vi "Demo - GNU Octave Terminal.vi"() -> ()   [LabVIEW 2013, in "GOLPI library.lvlib"]
uses:
  GOLPI library.lvlib
  LV Process.lvlibp/Pipe Handle.ctl
  LV Process.lvlibp
panel:
  out "bytes remaining":i32
  in  "quit":bool
  out "GNU Octave running":bool
  out "read buffer":string
  in  "command buffer":string
  in  "command":bool
  out "objects after start":refnum<vi>[](array[refnum])
  out "objects before start":refnum<vi>[](array[refnum])
  in  "stop":bool
  out "error":errorcluster
  out "octave pipe":T1
  in  "start":bool
  in  "Octave binary directory":path=path "C:/Program Files/Octave-3.6.2/bin"
  in  "Working directory":path=path "C:/"
  out "exit code":i32
  out "GNU Octave version":string
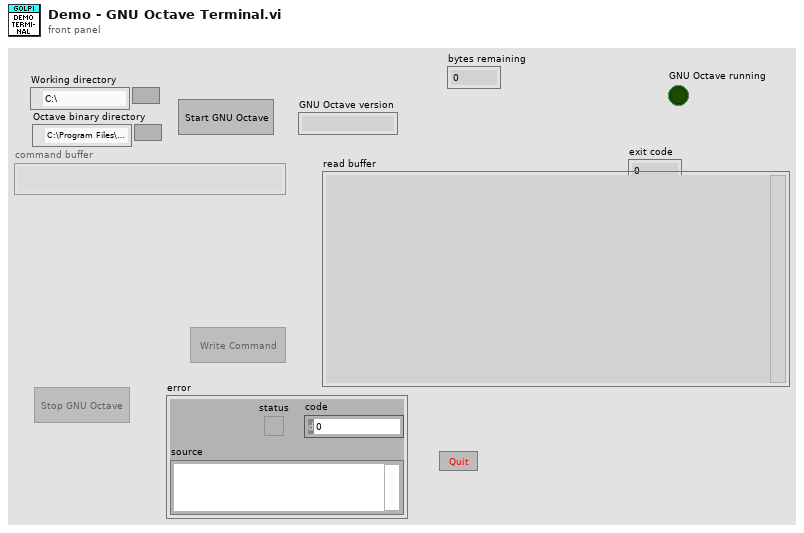
[diagram p1: front panel]
types:
  T1 = typedef "LV Process.lvlibp/Pipe Handle.ctl" = cluster{"lv_proc.dll file path":path, "process instance handle":u32[]}
  T2 = enum8{"Enabled", "Disabled", "Disabled and Grayed Out"}
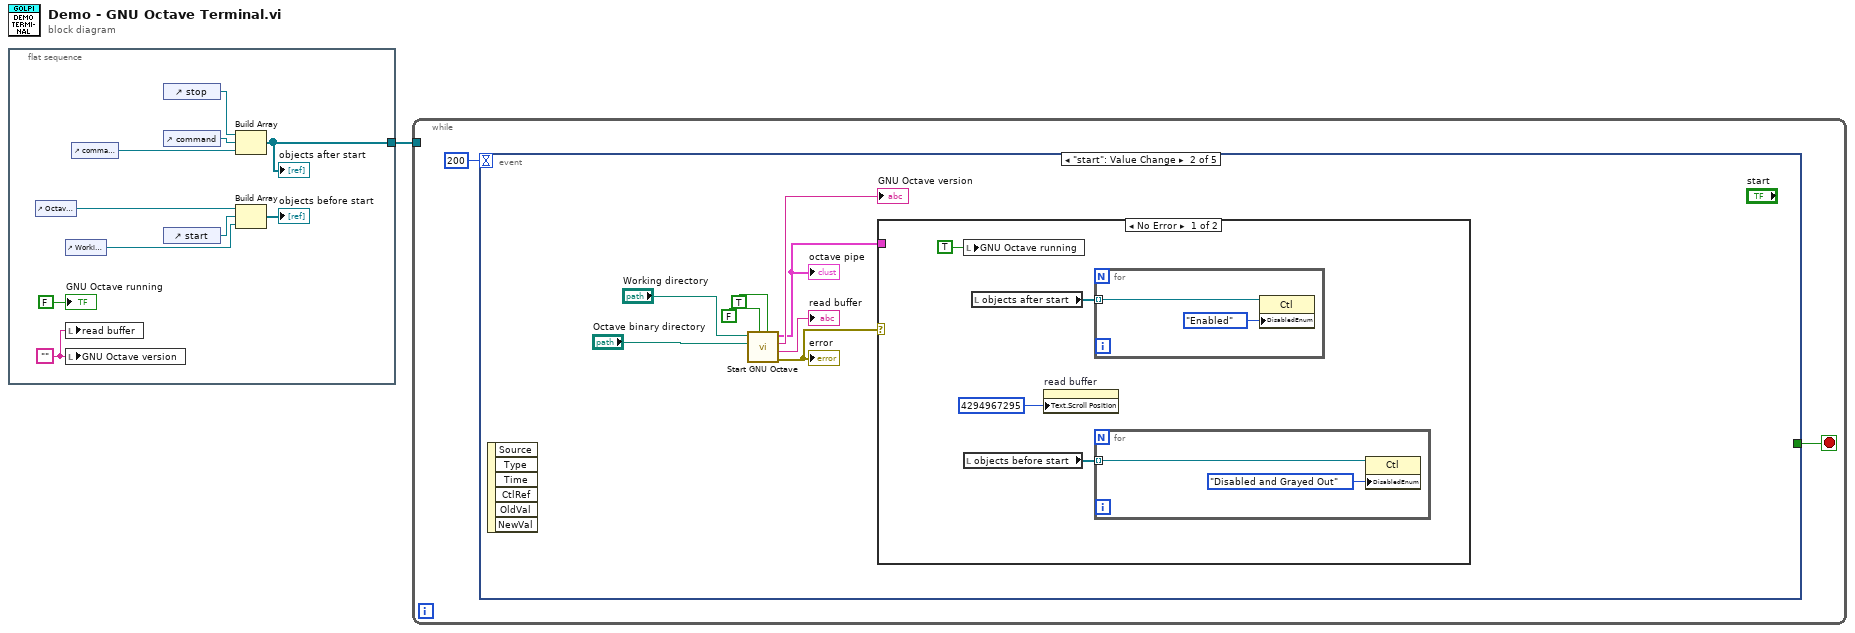
[diagram p0: block diagram]
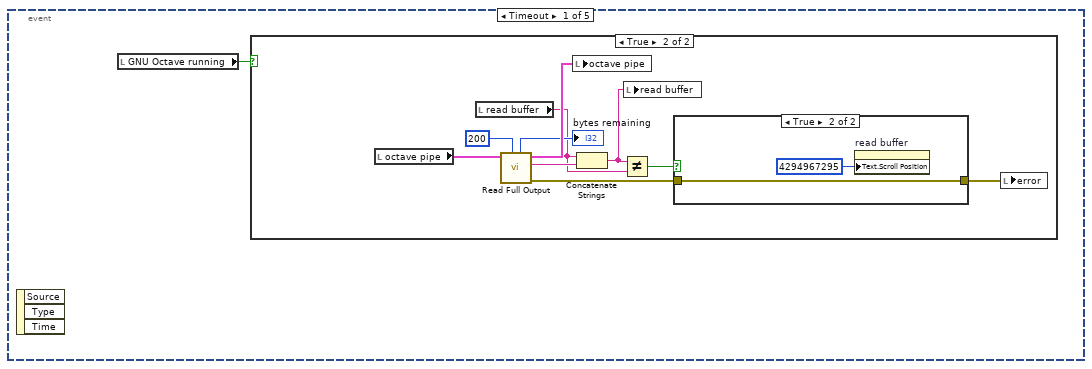
[diagram p2: hidden frame]
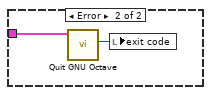
[diagram p5: hidden frame]
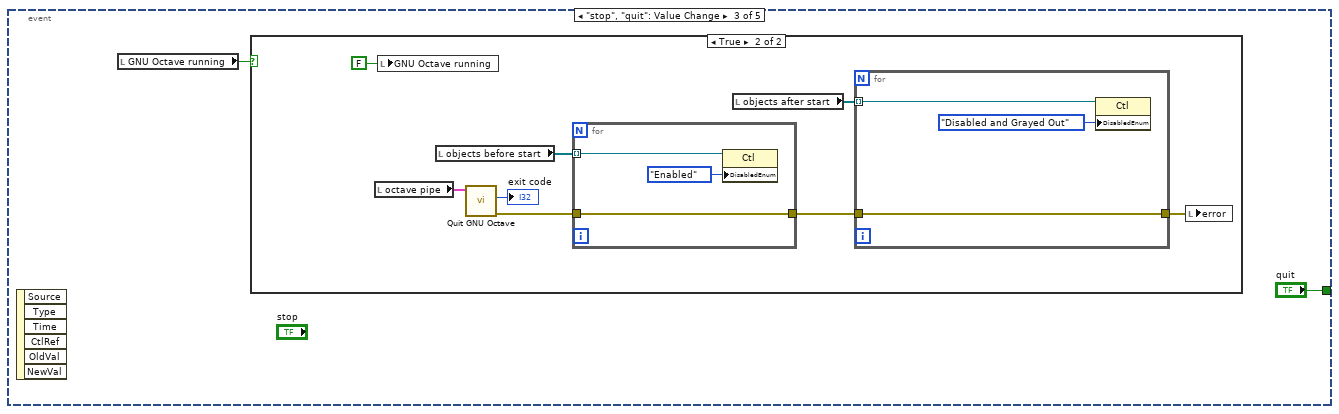
[diagram p6: hidden frame]
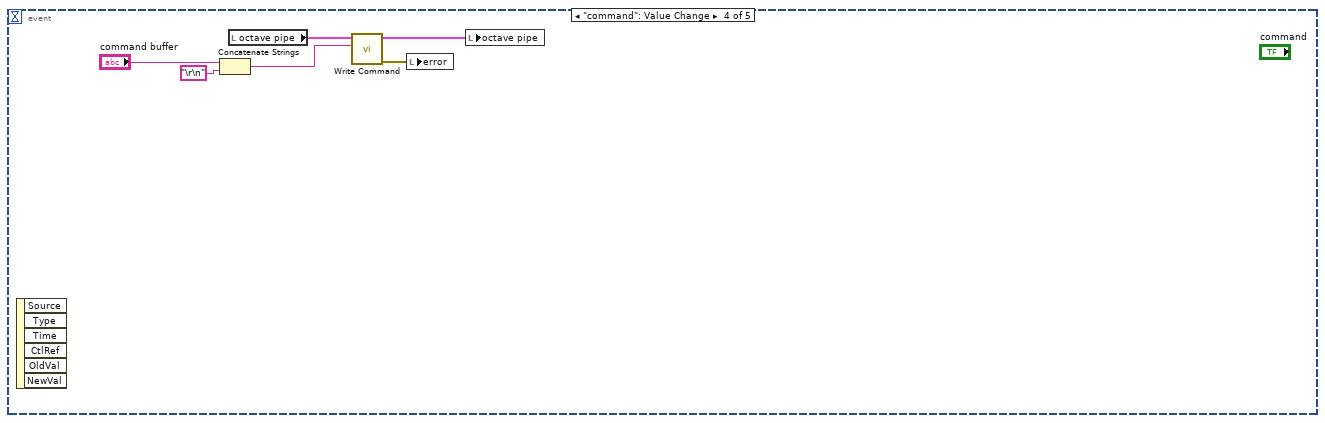
[diagram p8: hidden frame]
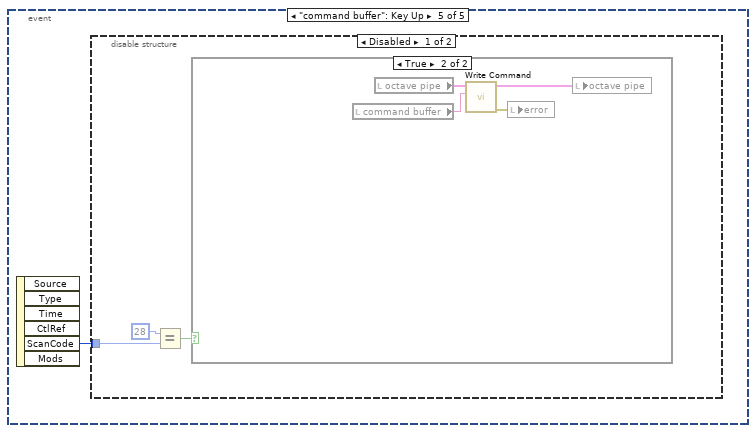
[diagram p9: hidden frame]
diagram:
  n1 = flat-sequence {
    tunnel: [w6] -> w1
    frame #0 {
      w3 = "" ("read buffer")
      n2 = control-ref of="Octave binary directory"() -> (w11:refnum<vi>)
      n3 = control-ref of="Working directory"() -> (w9:refnum<vi>)
      n4 = local write "read buffer"(w3) -> ()
      n5 = local write "GNU Octave version"(w3) -> ()
      n6 = control-ref of="command buffer"() -> (w4:refnum<vi>)
      n7 = control-ref of="stop"() -> (w7:refnum<vi>)
      n8 = control-ref of="command"() -> (w5:refnum<vi>)
      n9 = control-ref of="start"() -> (w10:refnum<vi>)
      n10 = Build Array(w7, w5, w4) -> (w6:refnum<vi>[])
      "objects after start" <- w6
      n11 = Build Array(w11, w10, w9) -> (→"objects before start":refnum<vi>[])
      "GNU Octave running" <- FALSE ("GNU Octave running")
    }
  }
  n12 = while {
    tunnel: w1 -> [_]
    stop <- w12 stop-if-true
    n13 = event shown="[1] \"start\": Value Change" {
      selector: _ -> [_ _ _ _ _]
      dyn-events: _ -> [_ _ _ _ _]
      timeout: 200 -> [_ _ _ _ _]
      tunnel: [_ _ "quit" _ _] -> w12
      event Timeout {
        n14 = event-data() -> ()  [unwired: 1 in, 3 out]
        n15 = local read "GNU Octave running"() -> (w14:bool)
        n16 = case shown="True" w14 {
          frame False {
          }
          frame True {
            n17 = local read "octave pipe"() -> (w23:T1)
            n18 = local read "read buffer"() -> (w16:string)
            n19 = call "Read Full Output.vi"("timeout [ms]"=u32 200, "pipe in"=w23) -> ("error out"=w21:errorcluster, "read buffer"=w22:string, "pipe out"=w20:T1, "bytes remaining"=→"bytes remaining":i32)  [unwired: 6 in]
            n20 = local write "octave pipe"(w20) -> ()
            n21 = Concatenate Strings(w16, w22) -> (w17:string)
            n22 = Not Equal?(x=w17, y=w16) -> (x != y?=w15:bool)
            n23 = local write "read buffer"(w17) -> ()
            n24 = case shown="True" w15 {
              tunnel: [w25 w26] -> w24
              tunnel: w21 -> [w25 w26]
              frame False {
              }
              frame True {
                n25 = property on="read buffer" class="Str"("Text.Scroll Position"=u32 4294967295) -> ()  [unwired: 2 in, 2 out]
              }
            }
            n26 = local write "error"(w24) -> ()
          }
        }
      }
      event "start": Value Change {
        n27 = event-data() -> ()  [unwired: 1 in, 6 out]
        n28 = call "Start GNU Octave.vi"(5:TRUE ("use stderr (F)"), 7:FALSE ("hide window (T)"), "Octave binary directory"="Octave binary directory", "Working directory"="Working directory") -> ("error out"=w32:errorcluster, "initial output"=→"read buffer":string, "GNU Octave version"=→"GNU Octave version":string, "pipe out"=w30:T1)  [unwired: 4 in]
        "octave pipe" <- w30
        "error" <- w32
        n29 = case shown="No Error" w32 {
          tunnel: w30 -> [_ w45]
          frame No Error {
            n30 = local write "GNU Octave running"(TRUE ("GNU Octave running")) -> ()
            n31 = local read "objects before start"() -> (w39:refnum<vi>[])
            n32 = local read "objects after start"() -> (w38:refnum<vi>[])
            n33 = property on="read buffer" class="Str"("Text.Scroll Position"=u32 4294967295) -> ()  [unwired: 2 in, 2 out]
            n34 = for {
              tunnel: w38 -> [w41] mode=indexing
              n35 = property class="Ctl"(reference=w41, "DisabledEnum"=T2."Enabled" ("Disabled")) -> ()  [unwired: 1 in, 2 out]
            }
            n36 = for {
              tunnel: w39 -> [w43] mode=indexing
              n37 = property class="Ctl"(reference=w43, "DisabledEnum"=T2."Disabled and Grayed Out" ("Disabled")) -> ()  [unwired: 1 in, 2 out]
            }
          }
          frame Error {
            n38 = call "Quit GNU Octave.vi"("pipe in"=w45) -> ("exit code"=w44:i32)  [unwired: 9 in, 1 out]
            n39 = local write "exit code"(w44) -> ()
          }
        }
      }
      event "stop", "quit": Value Change {
        n40 = event-data() -> ()  [unwired: 1 in, 6 out]
        n41 = local read "GNU Octave running"() -> (w46:bool)
        n42 = case shown="True" w46 {
          frame False {
          }
          frame True {
            n43 = local read "octave pipe"() -> (w51:T1)
            n44 = local write "GNU Octave running"(FALSE ("GNU Octave running")) -> ()
            n45 = local read "objects before start"() -> (w54:refnum<vi>[])
            n46 = call "Quit GNU Octave.vi"("pipe in"=w51) -> ("error out"=w50:errorcluster, "exit code"=→"exit code":i32)  [unwired: 9 in]
            n47 = for {
              tunnel: w54 -> [w61] mode=indexing
              tunnel: w50 -> [w59]
              tunnel: [w59] -> w49
              n48 = property class="Ctl"(reference=w61, "DisabledEnum"=T2."Enabled" ("Disabled")) -> ()  [unwired: 1 in, 2 out]
            }
            n49 = local read "objects after start"() -> (w53:refnum<vi>[])
            n50 = for {
              tunnel: w53 -> [w58] mode=indexing
              tunnel: [w56] -> w48
              tunnel: w49 -> [w56]
              n51 = property class="Ctl"(reference=w58, "DisabledEnum"=T2."Disabled and Grayed Out" ("Disabled")) -> ()  [unwired: 1 in, 2 out]
            }
            n52 = local write "error"(w48) -> ()
          }
        }
      }
      event "command": Value Change {
        n53 = event-data() -> ()  [unwired: 1 in, 6 out]
        n54 = Concatenate Strings("command buffer", "\r\n") -> (w62:string)
        n55 = local read "octave pipe"() -> (w67:T1)
        n56 = call "Write Command.vi"("command"=w62, "pipe in"=w67) -> ("error out"=w66:errorcluster, "pipe out"=w65:T1)  [unwired: 8 in]
        n57 = local write "error"(w66) -> ()
        n58 = local write "octave pipe"(w65) -> ()
      }
      event "command buffer": Key Up {
        n59 = event-data() -> ("ScanCode"=w68:i16)  [unwired: 1 in, 5 out]
        n60 = disable-structure shown="Disabled" {
          disable-tunnel: w68 -> [w70 _]
          frame Disabled {
            n61 = Equal?(x=i16 28, y=w70) -> (x = y?=w71:bool)
            n62 = case shown="True" w71 {
              frame False {
              }
              frame True {
                n63 = local read "command buffer"() -> (w75:string)
                n64 = local read "octave pipe"() -> (w72:T1)
                n65 = call "Write Command.vi"("command"=w75, "pipe in"=w72) -> ("error out"=w73:errorcluster, "pipe out"=w74:T1)  [unwired: 8 in]
                n66 = local write "error"(w73) -> ()
                n67 = local write "octave pipe"(w74) -> ()
              }
            }
          }
          frame Enabled {
          }
        }
      }
    }
  }
